vi "Error Write Watch.vi"(8 "error in":errorcluster, 10 "Watchdog STS":i32, 11 "Cycler in":refnum<class "Cycler.lvclass">) -> (0 "error out":errorcluster, 3 "Cycler out":refnum<class "Cycler.lvclass">)   [LabVIEW 2023, in "Cycler.lvclass"]
uses:
  Cycler.lvclass
  Cycler.lvclass/Cycler.ctl
  Low Level Capabilities/Error/Error.lvclass
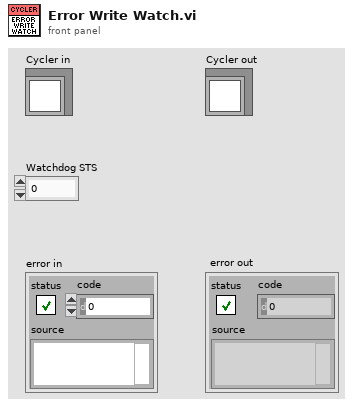
[diagram p1: front panel]
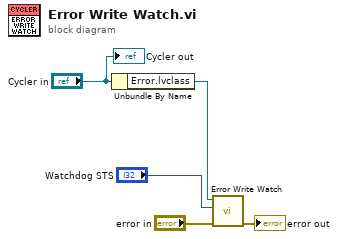
[diagram p0: block diagram]
diagram:
  n1 = Unbundle By Name("Cycler in") -> ("Error.lvclass"=w2:refnum<class "Error.lvclass">)
  n2 = call-dynamic "Error Write Watch.vi"("error in"="error in", "Watchdog STS"="Watchdog STS", "Error in"=w2) -> ("error out"=→"error out":errorcluster)  [unwired: 7 in, 1 out]
  "Cycler out" <- "Cycler in"
